vi "Init TCA9548A Mux.vi"(8 "error in (no error)":errorcluster, 10 "Address":u8=17 caption="(Default x11)" format="%.0x", 11 "TCA9548A Mux in":refnum<class "TCA9548A I2C Multiplexer.lvclass">) -> (0 "error out":errorcluster, 3 "TCA9548A Mux out":refnum<class "TCA9548A I2C Multiplexer.lvclass">)   [LabVIEW 2020, in "CTI-Peripheral.lvlib" / "TCA9548A I2C Multiplexer.lvclass"]
uses:
  TCA9548A I2C Multiplexer.lvclass
  TCA9548A I2C Multiplexer.lvclass/TCA9548A I2C Multiplexer.ctl
  CTI/I2C Connection/I2C Connection.lvclass/I2C Connection.ctl
  CTI/Session/I2C Write Data.vi
  CTI/I2C Connection/I2C Connection.lvclass
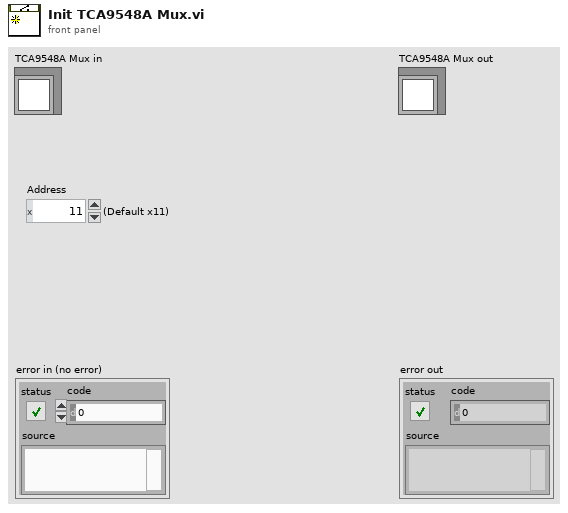
[diagram p1: front panel]
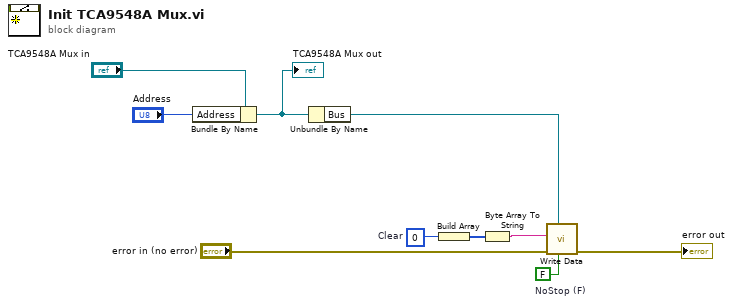
[diagram p0: block diagram]
diagram:
  w5 = u8 0  # Clear
  w6 = FALSE  # NoStop (F)
  n1 = Bundle By Name(cluster="TCA9548A Mux in", "Address"="Address") -> (w4:refnum<class "TCA9548A I2C Multiplexer.lvclass">)
  "TCA9548A Mux out" <- w4
  n2 = Unbundle By Name(w4) -> ("Bus"=w3:refnum<class "I2C Connection.lvclass">)
  n3 = Build Array(w5) -> (w8:u8[])
  n4 = Byte Array To String(unsigned byte array=w8) -> (string=w7:string)
  n5 = call "Write Data.vi"("NoStop (F)"=w6, "I2C Connection"=w3, "error in (no error)"="error in (no error)", "Data"=w7) -> ("error out"=→"error out":errorcluster)  [unwired: 7 in]
